vi "onConnection.vi"(8 "error in (no error)":errorcluster, 11 "Connection.TCP-TLS in":refnum<class "Connection.TCP-TLS.lvclass">) -> (0 "error out":errorcluster, 3 "Connection.TCP-TLS out":refnum<class "Connection.TCP-TLS.lvclass">)   [LabVIEW 2020, in "Connection.TCP-TLS.lvclass"]
uses:
  Connection.TCP-TLS.lvclass
  C:/Program Files (x86)/National Instruments/LabVIEW 2020/vi.lib/LabVIEW Open Source Project/MQTT Connection/MQTT_Connection/Connection/Connection.lvclass
  C:/Program Files (x86)/National Instruments/LabVIEW 2020/vi.lib/LabVIEW Open Source Project/MQTT TCP Connection/MQTT_TCP/Connection/TCPConnection.lvclass
  Connection.TCP-TLS.lvclass/Connection.TCP-TLS.ctl
  <vilib>/LabVIEW Open Source Project/MQTT Connection/MQTT_Connection/Connection/Connection.lvclass/Connection.ctl
  <vilib>/LabVIEW Open Source Project/MQTT Connection/MQTT_Connection/Connection/Connection.lvclass
  <vilib>/LabVIEW Open Source Project/MQTT TCP Connection/MQTT_TCP/Connection/TCPConnection.lvclass
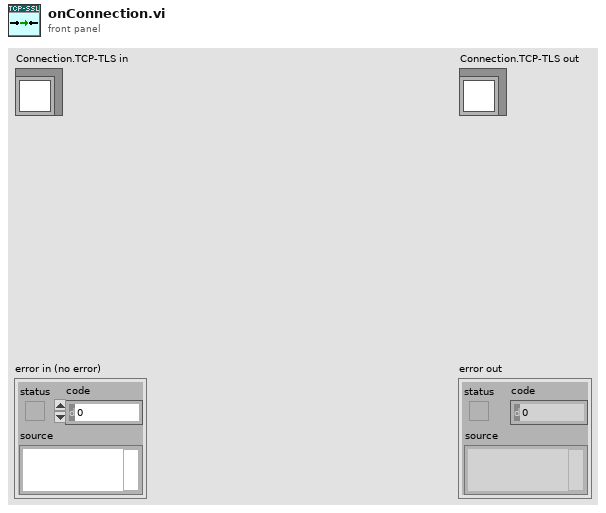
[diagram p1: front panel]
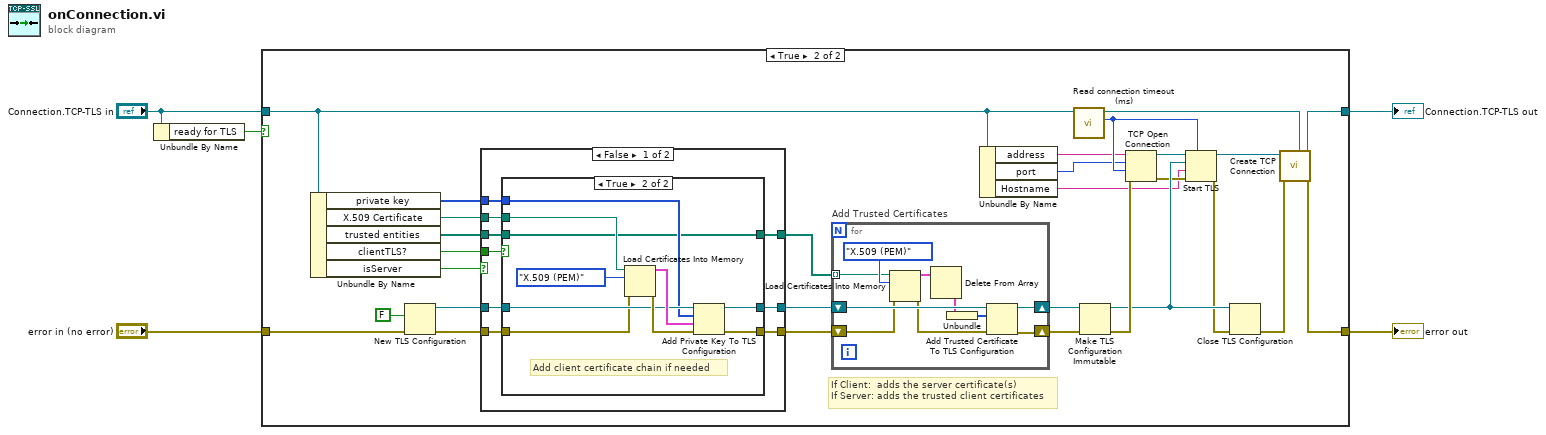
[diagram p0: block diagram]
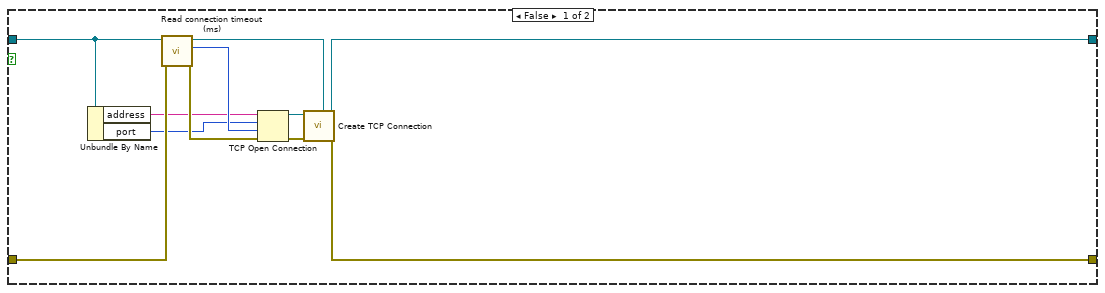
[diagram p2: hidden frame]
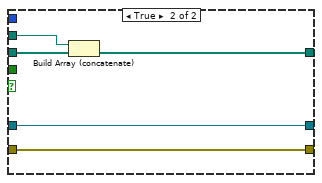
[diagram p4: hidden frame]
diagram:
  n1 = Unbundle By Name("Connection.TCP-TLS in") -> ("ready for TLS"=w4:bool)
  n2 = case shown="True" w4 {
    tunnel: "Connection.TCP-TLS in" -> [w13 w42]
    tunnel: [w8 w43] -> w2
    tunnel: "error in (no error)" -> [w15 w45]
    tunnel: [w6 w44] -> w1
    frame False {
      n3 = Unbundle By Name(w13) -> ("address"=w12:string, "port"=w11:u16)
      n4 = call <vilib>:"Read connection timeout (ms).vi"("error in (no error)"=w15, "Connection in"=w13) -> ("error out"=w14:errorcluster, "connection timeout (ms)"=w16:i32, "Connection out"=w9:refnum<class "Connection.TCP-TLS.lvclass">)  [unwired: 7 in]
      n5 = TCP Open Connection(address=w12, remote port or service name=w11, timeout ms (60000)=w16, error in (no error)=w14) -> (connection ID=w10:refnum<k5>, error out=w7:errorcluster)  [unwired: 1 in]
      n6 = call <vilib>:"Create TCP Connection.vi"("TCPConnection in"=w9, "error in (no error)"=w7, "connection ID"=w10) -> ("error out"=w6:errorcluster, "TCPConnection out"=w8:refnum<class "Connection.TCP-TLS.lvclass">)  [unwired: 7 in]
    }
    frame True {
      # "If Client:  adds the server certificate(s)\nIf Server: adds the trusted client certificates"
      n7 = Unbundle By Name(w42) -> ("private key"=w20:u8[], "X.509 Certificate"=w25:path, "trusted entities"=w24:path[], "clientTLS?"=w18:bool, "isServer"=w19:bool)
      n8 = New TLS Configuration(8:w45, 10:FALSE ("load OS trusted CAs?")) -> (0:w40:errorcluster, 3:w39:refnum<k36>)
      n9 = case shown="False" w19 {
        tunnel: w25 -> [w50 w70]
        tunnel: w24 -> [w46 w68]
        tunnel: [w47 w69] -> w23
        tunnel: [w54 w72] -> w22
        tunnel: w39 -> [w53 w72]
        tunnel: [w52 w71] -> w21
        tunnel: w40 -> [w51 w71]
        tunnel: w20 -> [w49 _]
        tunnel: w18 -> [w48 _]
        frame False {
          n10 = case shown="True" w48 {
            tunnel: [w56 w64] -> w54
            tunnel: w53 -> [w56 w63]
            tunnel: [w55 w62] -> w52
            tunnel: w51 -> [w55 w61]
            tunnel: w50 -> [_ w60]
            tunnel: w49 -> [_ w59]
            tunnel: [w57 w58] -> w47
            tunnel: w46 -> [w57 w58]
            frame False {
            }
            frame True {
              # "Add client certificate chain if needed"
              n11 = Load Certificates Into Memory(8:w61, 10:enum32{"X.509 (PEM)"}."X.509 (PEM)" ("format"), 11:w60) -> (0:w66:errorcluster, 3:w67:cluster{"certificate":u8[]}[])
              n12 = Add Private Key To TLS Configuration(8:w66, 9:w67, 10:w59, 11:w63) -> (0:w62:errorcluster, 3:w64:refnum<k36>)
            }
          }
        }
        frame True {
          n13 = Build Array (concatenate)(w70, w68) -> (w69:path[])
        }
      }
      n14 = for "Add Trusted Certificates" {
        shift-right: [w80] -> w29
        shift-left: w21 -> [w77]
        shift-right: [w79] -> w30
        shift-left: w22 -> [w81]
        tunnel: w23 -> [w73] mode=indexing
        n15 = Load Certificates Into Memory(8:w77, 10:enum32{"X.509 (PEM)"}."X.509 (PEM)" ("format"), 11:w73) -> (0:w78:errorcluster, 3:w75:cluster{"certificate":u8[]}[])
        n16 = Delete From Array(array=w75) -> (deleted portion=w74:cluster{"certificate":u8[]})  [unwired: 2 in, 1 out]
        n17 = Unbundle(w74) -> ("certificate"=w76:u8[])
        n18 = Add Trusted Certificate To TLS Configuration(8:w78, 10:w76, 11:w81) -> (0:w80:errorcluster, 3:w79:refnum<k36>)
      }
      n19 = Unbundle By Name(w42) -> ("address"=w28:string, "port"=w27:u16, "Hostname"=w26:string)
      n20 = call <vilib>:"Read connection timeout (ms).vi"("Connection in"=w42) -> ("connection timeout (ms)"=w35:i32, "Connection out"=w32:refnum<class "Connection.TCP-TLS.lvclass">)  [unwired: 8 in, 1 out]
      n21 = Make TLS Configuration Immutable(8:w29, 11:w30) -> (0:w38:errorcluster, 3:w36:refnum<k36>)
      n22 = TCP Open Connection(address=w28, remote port or service name=w27, timeout ms (60000)=w35, error in (no error)=w38) -> (connection ID=w37:refnum<k5>, error out=w34:errorcluster)  [unwired: 1 in]
      n23 = Start TLS(7:w35, 8:w34, 9:w26, 10:w36, 11:w37) -> (0:w33:errorcluster, 3:w17:refnum<k5>)  [unwired: 1 in, 1 out]
      n24 = Close TLS Configuration(8:w33, 11:w36) -> (0:w31:errorcluster)
      n25 = call <vilib>:"Create TCP Connection.vi"("TCPConnection in"=w32, "error in (no error)"=w31, "connection ID"=w17) -> ("error out"=w44:errorcluster, "TCPConnection out"=w43:refnum<class "Connection.TCP-TLS.lvclass">)  [unwired: 7 in]
    }
  }
  "error out" <- w1
  "Connection.TCP-TLS out" <- w2
